vi "Dashboard Main.vi"() -> ()   [LabVIEW 2018]
uses:
  <vilib>/Utility/miscctls.llb/LVRowAndColumnTypeDef.ctl
  <vilib>/event_ctls.llb/eventvkey.ctl
  <vilib>/Rock Robotics/Network Tables/NT Read Numeric Array.vi
  <vilib>/Rock Robotics/Network Tables/NT Write Boolean.vi
  <vilib>/Rock Robotics/Network Tables/NT Read Boolean.vi
  <vilib>/Rock Robotics/WPI/Dashboard/WPI_DashboardLogging Global.vi
panel:
  in  "Camera Settings Right":T1={"Frame Rate"=30, "Compression"=30, "Size"=1, "DB Camera Config"=FALSE} {"Frame Rate" scale=1.0..30.0; "Compression" scale=100.0..-1.0; "Size" items=["640x480", "320x240", "160x120"]}
  in  "Camera Name Right":string(combo)="No Camera Selection"
  out "Camera Perf":string
  in  "Camera Settings":T1={"Frame Rate"=30, "Compression"=30, "Size"=1, "DB Camera Config"=FALSE} {"Frame Rate" scale=1.0..30.0; "Compression" scale=100.0..-1.0; "Size" items=["640x480", "320x240", "160x120"]}
  in  "TCP":refnum<k5>
  in  "Rec Mode":enum32{"Stop", "Record", "Playback"}(radio)
  out "Robot IP":string
  out "Image Message":string="Timeout in Camera Communications"
  in  "Dashboard Tab":T2(tab)
  in  "Select Auto":string(combo)="Select Autonomous ..."
  out "NT Connection":bool
  out "MotorChart R":cluster{"Numeric":dbl, "Numeric":dbl}(graph)
  out "MotorChart L":cluster{"Numeric":dbl, "Numeric":dbl}(graph)
  out "MotorSliders R":cluster{"MotorSlide1":dbl, "MotorSlide2":dbl} {"MotorSlide2" scale=-1.0..1.0 scale format="%#_2e"; "MotorSlide1" scale=-1.0..1.0 scale format="%#_2e"}
  out "MotorSliders L":cluster{"MotorSlide1":dbl, "MotorSlide2":dbl} {"MotorSlide2" scale=-1.0..1.0 scale format="%#_2e"; "MotorSlide1" scale=-1.0..1.0 scale format="%#_2e"}
  out "Gyro":dbl(knob) scale=0.0..360.0
  out "JS1 Z":dbl(slide) scale=-1.0..1.0 scale format="%#_2e"
  out "JS1 Graph":cluster{"X":dbl, "Y":dbl}[](graph)
  out "JS1 Buttons":T3
  out "JS2 Z":dbl(slide) scale=-1.0..1.0 scale format="%#_2e"
  out "JS2 Graph":cluster{"X":dbl, "Y":dbl}[](graph)
  out "JS2 Buttons":T3
  out "Mode":T4(ring)=enum."Auto Disabled"
  out "Right Camera Perf":cluster{"Bandwidth (Mbps)":dbl, "FPS":dbl}
  out "Camera Image Right":T5(plugin-control)
  in  "DB/String 9":string
  in  "DB/String 8":string
  in  "DB/String 7":string
  in  "DB/String 6":string
  in  "DB/String 5":string
  in  "DB/String 4":string
  in  "DB/String 3":string
  in  "DB/String 2":string
  in  "DB/String 1":string
  in  "DB/String 0":string
  in  "DB/Slider 0":dbl(slide) scale=0.0..5.0
  in  "DB/Slider 1":dbl(slide) scale=0.0..5.0
  in  "DB/Slider 2":dbl(slide) scale=0.0..5.0
  in  "DB/Slider 3":dbl(slide) scale=0.0..5.0
  out "DB/LED 3":bool
  out "DB/LED 2":bool
  out "DB/LED 1":bool
  out "DB/LED 0":bool
  in  "DB/Button 3":bool
  in  "DB/Button 2":bool
  in  "DB/Button 1":bool
  in  "DB/Button 0":bool caption="New Name"
  in  "Robot Front":bool
  in  "Calibrate?":bool
  out "ElevEncPos":dbl
  out "ElevBasePos":string
  out "PickUp/DropOff":string
  out "SwerveMode":string
  out "Yaw":dbl
  out "Hatch Position":bool
  in  "Test Slider":dbl(slide) scale=0.0..100.0 scale format="%#_3g"
  in  "On/Off":bool caption="Solenoid"
  in  "Test Name":u16(ring) items=["Select the test to run..."]
  in  "Test Tree":string(tree)
  in  "Motor":cluster{"Value":dbl, "Enable":bool} {"Value" scale=-1.0..1.0 scale format="%#_3g"}
  out "Progress":T6 {"Test Progress" scale=0.0..100.0}
  in  "Rev/Fwd":cluster{"Forward":bool, "Reverse":bool}
  in  "Test Ring":u16(ring) items=["Monochrome", "Color"]
  out "Cmd Status":string
  in  "Execute Command":bool
  in  "Command Params":string[][](table)
  in  "Command Selection":i32(listbox)
  in  "CheckList":i32(listbox)
  out "Tree":string(tree)
  out "Camera Image":T5(plugin-control)
  out "Background":bool
  in  "Camera Name":string(combo)="No Camera Selection"
  # "HW"
  # "HW"
  # "Joysticks"
  # "Drive Motors"
  # "Front"
  # "Right"
  # "Left"
  # "Back"
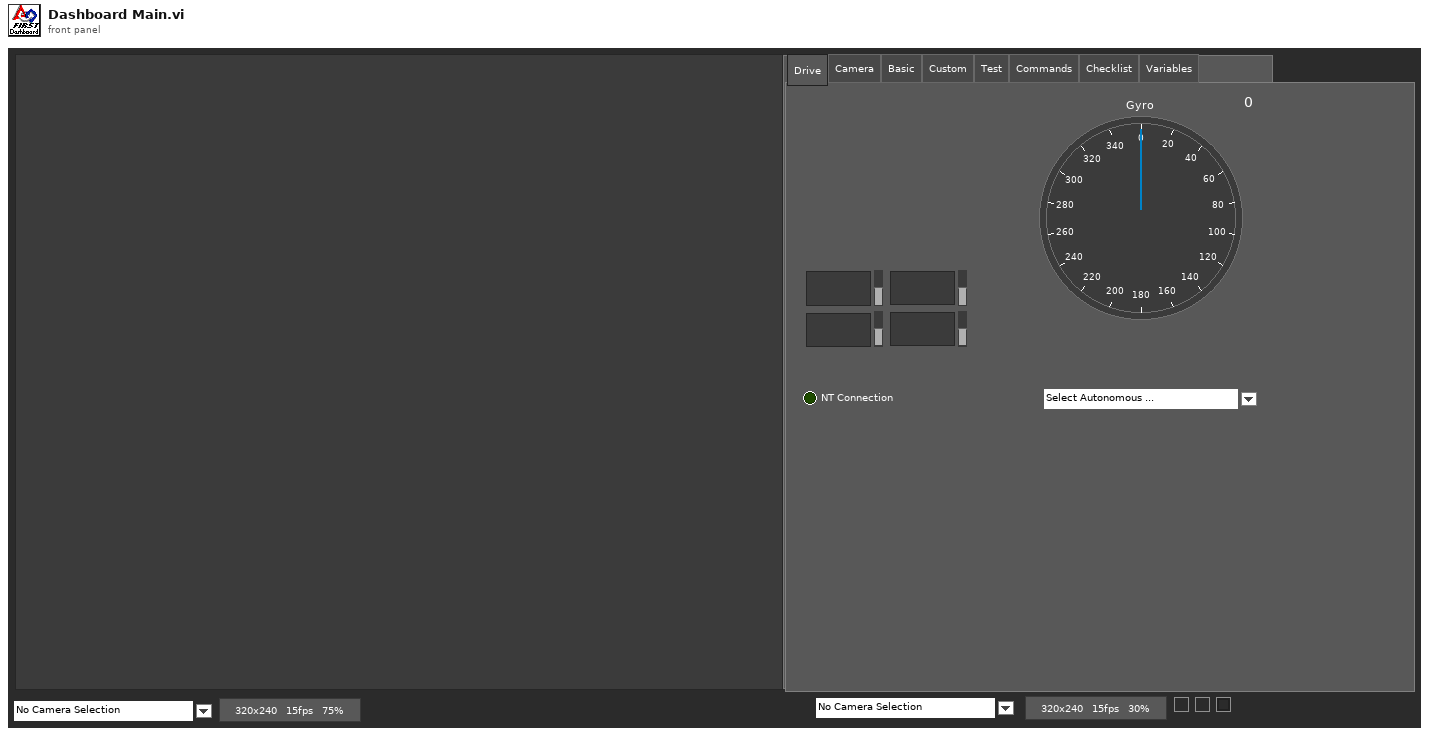
[diagram p1: front panel]
types:
  T1 = cluster{"Frame Rate":i32, "Compression":i32, "Size":u16, "DB Camera Config":bool}
  T2 = enum32{"Drive", "Camera", "Basic", "Custom", "Test", "Commands", "Checklist", "Variables"}
  T3 = cluster{bool, bool, bool, bool, bool, bool, bool, bool, bool, bool, bool, bool}
  T4 = enum8{"Tele-Op Disabled", "Tele-Op Enabled", "Auto Disabled", "Auto Enabled", "Test Disabled", "Test Enabled", "Disconnected", "No Code", "E-Stop"}
  T5 = typedef "IMAQ Image.ctl" = refnum<image>
  T6 = cluster{"Test Progress":u8, "Test Progress Text":string}
  T7 = cluster{"Save Path":path, "Interval (s)":dbl, "Keep":i32}
  T8 = typedef "Image Type" = u32
  T9 = cluster{"IDs":cluster{"RPC field ID":u16, "Unique ID":u16}, "String":string}
  T10 = cluster{"Error Strings":string, "Disable Counts":cluster{u16, u16}, "Rail Faults":cluster{u16, u16, u16}, "Robot IP":string, "DB Mode":u8, "Event Info":cluster{"Name":string, "Type":u8, "Number":u16, "Replay":u8}}
  T11 = cluster{"Storage":cluster{"Disk Free":u64, "RAM Block":u32, "RAM free":u32}, "CPU Utilization":cluster{"CPU % ISR":sgl, "CPU % Time Crit":sgl, "CPU % Timed Str":sgl, "CPU % High":sgl, "CPU % Above":sgl, "CPU % Normal":sgl, "CPU % Low":sgl}, "CAN":cluster{"% Bus Utilization":sgl, "Bus Off Cnt":u32, "TX_FIFO Full Cnt":u32, "Receive Error Cnt":u8, "Transmit Error Cnt":u8}, "HID":cluster{"HID Outputs":u32, "Rumble Low":u16, "Rumble High":u16}[]}
  T12 = cluster{"Status bits":cluster{"Test Mode":bool, "Autonomous":bool, "Enabled":bool, "Code Start":bool, "Brownout":bool, "Reserved 2":bool, "Reserved 3":bool, "E-Stop":bool}, "Code Trace":cluster{"Disabled":bool, "TeleOp":bool, "Auto":bool, "Test":bool}, "Controller Type":enum16{"unknown", "cRIO", "roboRio"}, "Code?":enum16{"unknown", "noCode", "code"}, "Battery V":dbl}
  T13 = cluster{"Control Bits":cluster{"TestMode":bool, "Autonomous":bool, "Enabled":bool, "FMS Present":bool, bool, bool, bool, "E-Stop":bool}, "Team Station ":u8, "Countdown":sgl, "Joystick Values":cluster{"Axes":dbl[], "Buttons":bool[], "POVs":i16[]}[]}
  T14 = cluster{"Axes":dbl[], "Buttons":bool[], "POVs":i16[]}[]
  T15 = cluster{"Axes":dbl[], "Buttons":bool[], "POVs":i16[]}
  T16 = cluster{"Buttons[0]":bool, "Buttons[1]":bool, "Buttons[2]":bool, "Buttons[3]":bool, "Buttons[4]":bool, "Buttons[5]":bool, "Buttons[6]":bool, "Buttons[7]":bool, "Buttons[8]":bool, "Buttons[9]":bool, "Buttons[10]":bool, "Buttons[11]":bool}
  T17 = cluster{"Camera Image":refnum<vi>, "Dashboard Tab":refnum<vi>, "Background":refnum<vi>, "Rec Mode":refnum<vi>, "Test Slider":refnum<vi>, "On/Off ":refnum<vi>, "Test Ring":refnum<vi>, "Rev/Fwd":refnum<vi>, "Test Name":refnum<vi>, "Motor":refnum<vi>, "Progress":refnum<vi>, "CheckList":refnum<vi>, "Tree":refnum<vi>, "Test Tree":refnum<vi>, "Command Params":refnum<vi>, "Command Selection":refnum<vi>, "Execute Command":refnum<vi>, "Cmd Status":refnum<vi>, "Camera Settings":refnum<vi>, "Camera Name":refnum<vi>, "Camera Perf":refnum<vi>, "Camera Settings Right":refnum<vi>, "Camera Name Right":refnum<vi>, "Camera Image Right":refnum<vi>}
  T18 = cluster{"Global Rectangle":i32[], "Contours":cluster{"Contour Type":u32, "ROI Type":u32, "Points":i32[]}[]}
  T19 = cluster{"Camera Name":string, string, "Saved DB Images Info":cluster{"Save Path":path, "Interval (s)":dbl, "Keep":i32}}
  T20 = cluster{"Camera Name Right":string, string, "Saved DB Images Info":cluster{"Save Path":path, "Interval (s)":dbl, "Keep":i32}}
  T21 = cluster{"Operation":enum16{"Update", "Clear"}, "Color Box":u32}[]
  T22 = typedef "eventvkey.ctl" = enum16{"ASCII", "Enter", "Return", "Shift", "Ctrl", "Alt", "Cmd", "Opt", "Caps", "NumLock", "Clear", "Break", "Up", "Down", "Left", "Right", "Insert", "Delete", "Home", "End", "PageUp", "PageDown", "Escape", "Help", "Pause", "ScrollLock", "F1", "F2", "F3", "F4", "F5", "F6", "F7", "F8", "F9", "F10", "F11", "F12", "F13", "F14", "F15", "F16", "F17", "F18", "F19", "F20", "F21", "F22", "F23", "F24", "Play", "VolumeUp", "VolumeDown", "Mute", "Two Byte Char"}
  T23 = cluster{"Image Size":bool, "Image Type":bool, "Pixel Value":bool, "ROI Information":bool, "Zoom Factor":bool}
  T24 = cluster{"Operation":enum16{"Update", "Clear"}, "Color Box":u32}
  T25 = typedef "LVRowAndColumnTypeDef.ctl" = cluster{"Row":i32, "Column":i32}
  T26 = cluster{"Shift":bool, "Ctrl":bool, "Alt":bool, "Cmd":bool, "Opt":bool}
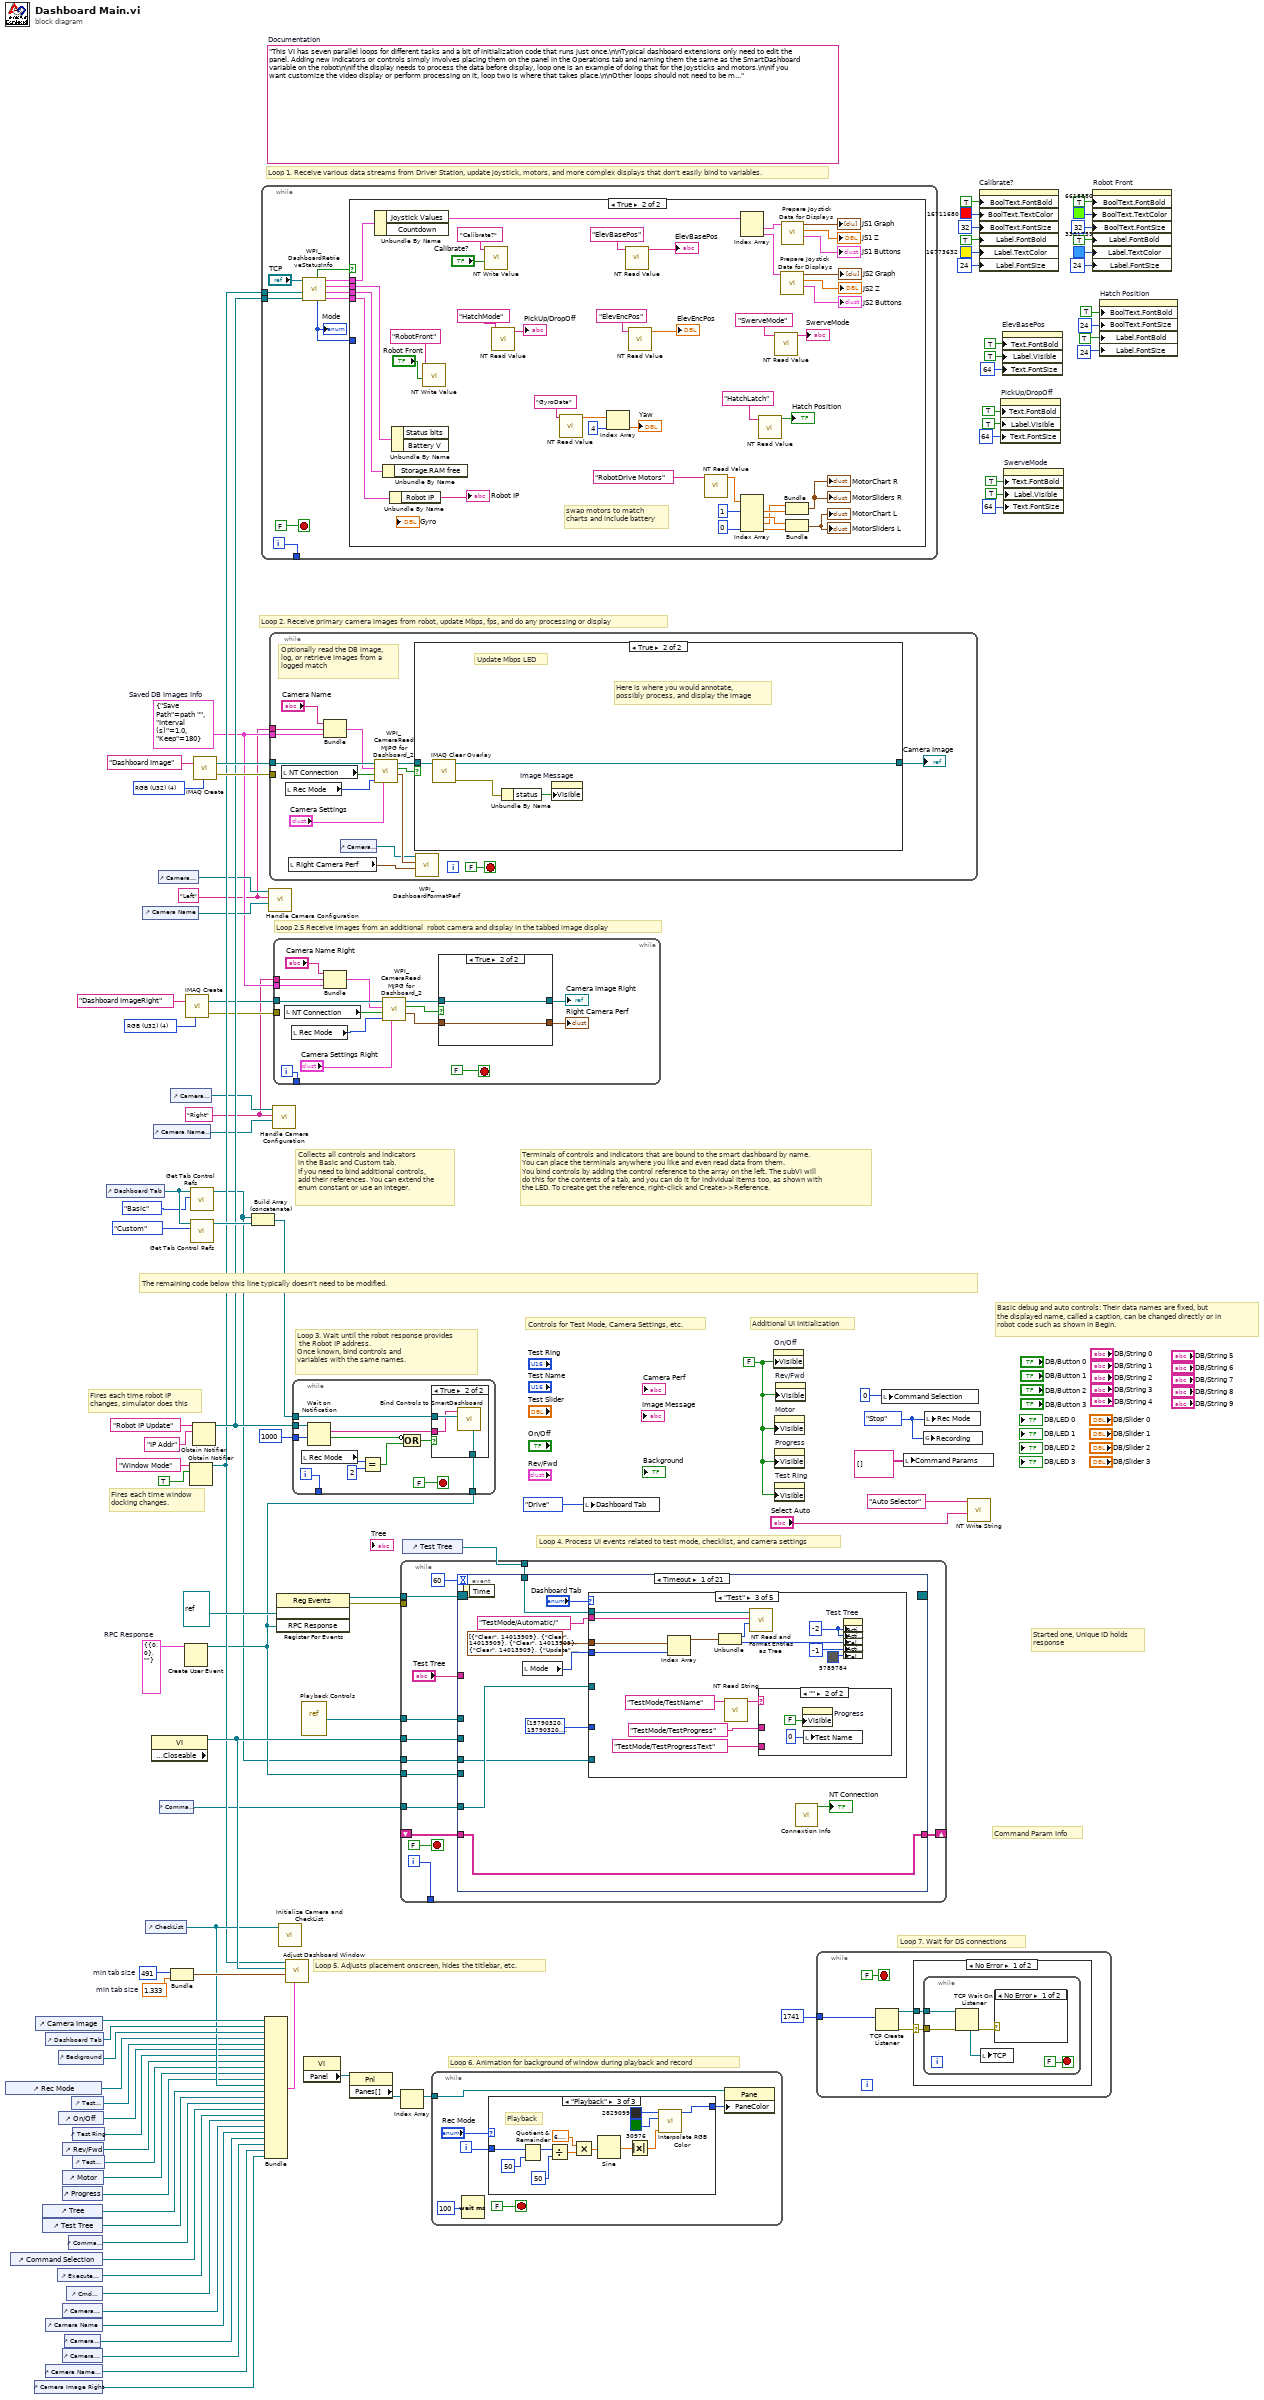
[diagram p0: block diagram]
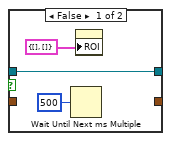
[diagram p2: hidden frame]
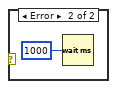
[diagram p3: hidden frame]
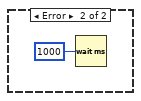
[diagram p4: hidden frame]
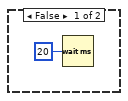
[diagram p5: hidden frame]
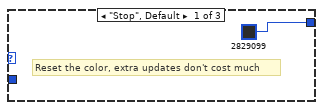
[diagram p6: hidden frame]
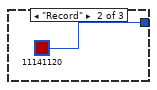
[diagram p7: hidden frame]
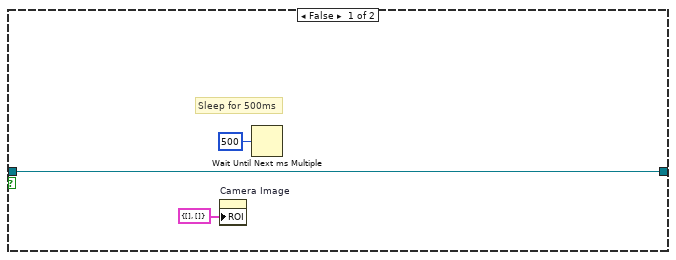
[diagram p9: hidden frame]
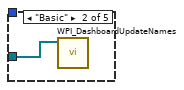
[diagram p11: hidden frame]
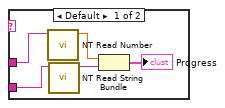
[diagram p12: hidden frame]
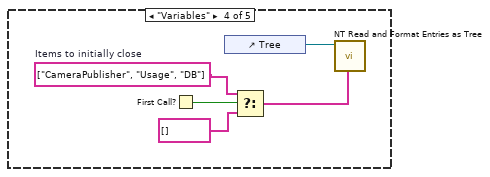
[diagram p13: hidden frame]
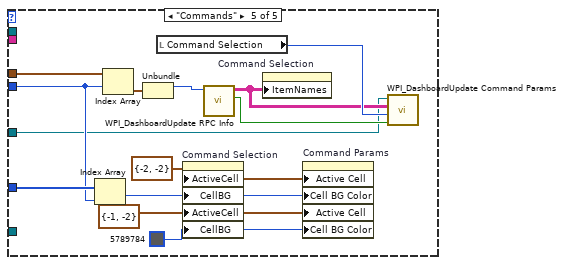
[diagram p14: hidden frame]
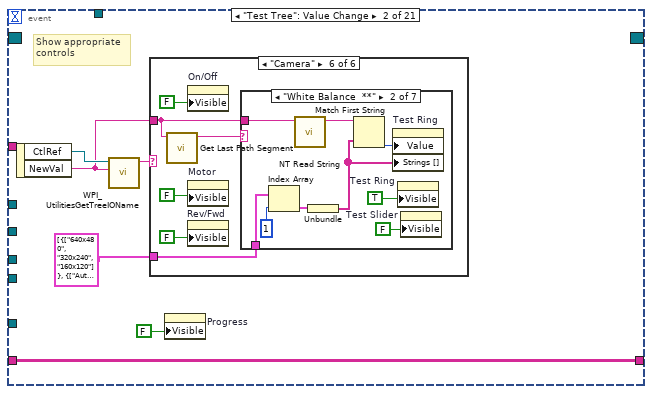
[diagram p15: hidden frame]
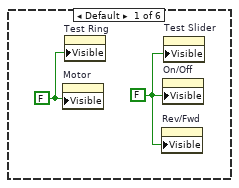
[diagram p16: hidden frame]
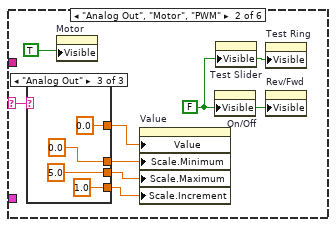
[diagram p17: hidden frame]
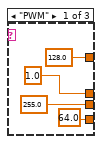
[diagram p18: hidden frame]
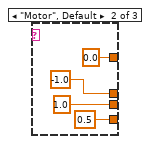
[diagram p19: hidden frame]
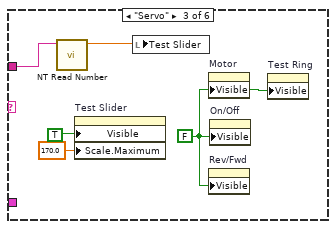
[diagram p20: hidden frame]
diagram:
  w28 = T7 {"Save Path"=path "", "Interval (s)"=1.0, "Keep"=180}  # Saved DB Images Info
  w27 = "Right"
  w26 = "Left"
  w38 = T8 4 items=["Grayscale (U8)", "Grayscale (I16)", "Grayscale (SGL)", "Complex (CSG)", "RGB (U32)", "HSL (U32)", "RGB (U64)"] ("Image Type")
  w54 = T9 {"IDs"={"RPC field ID"=0, "Unique ID"=0}, "String"=""}  # RPC Response
  w77 = 491  # min tab size
  w76 = 1.333  # min tab size
  w84 = enum32{"Stop", "Record", "Playback"}."Stop" ("Rec Mode")
  w61 = FALSE ("Visible")
  (unwired) "This VI has seven parallel loops for different tasks and a bit of initialization code that runs just once.\n\nTypical dashboard extensions only need to edit the panel. Adding new indicators or controls simply involves placing them on the panel in the Operations tab and naming them the same as the SmartDashboard variable on the robot\n\nIf the display needs to process the data before display, loop one is an example of doing that for the joysticks and motors.\n\nIf you want customize the video display or perform processing on it, loop two is where that takes place.\n\nOther loops should not need to be modified. They are pretty standard, and document the task they perform."  # Documentation
  w101 = T8 4 items=["Grayscale (U8)", "Grayscale (I16)", "Grayscale (SGL)", "Complex (CSG)", "RGB (U32)", "HSL (U32)", "RGB (U64)"] ("Image Type")
  # "Loop 2.5 Receive images from an additional  robot camera and display in the tabbed image display"
  # "Command Param Info"
  # "Started one, Unique ID holds\nresponse"
  # "Loop 7. Wait for DS connections"
  # "Basic debug and auto controls: Their data names are fixed, but\nthe displayed name, called a caption, can be changed directly or in\nrobot code such as shown in Begin."
  # "Controls for Test Mode, Camera Settings, etc."
  # "Additional UI Initialization"
  # "Loop 6. Animation for background of window during playback and record"
  # "Fires each time robot IP\nchanges, simulator does this"
  # "Fires each time window\ndocking changes."
  # "Collects all controls and indicators\nin the Basic and Custom tab.\nIf you need to bind additional controls,\nadd their references. You can extend the\nenum constant or use an integer."
  # "The remaining code below this line typically doesn't need to be modified."
  # "Loop 4. Process UI events related to test mode, checklist, and camera settings"
  # "Terminals of controls and indicators that are bound to the smart dashboard by name.\nYou can place the terminals anywhere you like and even read data from them.\nYou bind controls by adding the control reference to the array on the left. The subVI will\ndo this for the contents of a tab, and you can do it for individual items too, as shown with\nthe LED. To create get the reference, right-click and Create>>Reference."
  # "Loop 3. Wait until the robot response provides\n the Robot IP address.\nOnce known, bind controls and\nvariables with the same names."
  # "Loop 5. Adjusts placement onscreen, hides the titlebar, etc."
  # "Loop 1. Receive various data streams from Driver Station, update joystick, motors, and more complex displays that don't easily bind to variables."
  # "Loop 2. Receive primary camera images from robot, update Mbps, fps, and do any processing or display"
  n1 = control-ref of="Rec Mode"() -> (w67:refnum<vi>)
  n2 = control-ref of="Command Selection"() -> (w53:refnum<vi>)
  n3 = control-ref of="Camera Image Right"() -> (w31:refnum<vi>)
  n4 = control-ref of="Camera Image"() -> (w79:refnum<vi>)
  n5 = control-ref of="Tree"() -> (w71:refnum<vi>)
  n6 = control-ref of="Test Tree"() -> (w70:refnum<vi>)
  n7 = control-ref of="Dashboard Tab"() -> (w78:refnum<vi>)
  n8 = control-ref of="Camera Name"() -> (w44:refnum<vi>)
  n9 = control-ref of="Camera Name Right"() -> (w32:refnum<vi>)
  n10 = control-ref of="Execute Command"() -> (w55:refnum<vi>)
  n11 = control-ref of="Background"() -> (w74:refnum<vi>)
  n12 = control-ref of="On/Off"() -> (w65:refnum<vi>)
  n13 = control-ref of="Progress"() -> (w62:refnum<vi>)
  n14 = control-ref of="Camera Settings"() -> (w45:refnum<vi>)
  n15 = control-ref of="Camera Settings Right"() -> (w33:refnum<vi>)
  n16 = control-ref of="Rev/Fwd"() -> (w63:refnum<vi>)
  n17 = control-ref of="Motor"() -> (w68:refnum<vi>)
  n18 = control-ref of="Camera Perf"() -> (w43:refnum<vi>)
  n19 = control-ref of="Cmd Status"() -> (w49:refnum<vi>)
  n20 = control-ref of="Command Params"() -> (w56:refnum<vi>)
  n21 = control-ref of="Test Slider"() -> (w66:refnum<vi>)
  n22 = control-ref of="Test Ring"() -> (w64:refnum<vi>)
  n23 = control-ref of="Test Name"() -> (w69:refnum<vi>)
  n24 = control-ref of="Dashboard Tab"() -> (w82:refnum<vi>)
  n25 = control-ref of="Camera Name"() -> (w46:refnum<vi>)
  n26 = control-ref of="CheckList"() -> (w72:refnum<vi>)
  n27 = property class="VI" props=["Front Panel.Closeable"]() -> (reference out=w83:refnum<vi>)  [unwired: 2 in, 2 out]
  n28 = control-ref of="Camera Name Right"() -> (w34:refnum<vi>)
  n29 = control-ref of="Camera Settings"() -> (w47:refnum<vi>)
  n30 = control-ref of="Command Params"() -> (w48:refnum<vi>)
  n31 = control-ref of="Camera Settings Right"() -> (w35:refnum<vi>)
  n32 = Bundle("min tab size"=w77, "min tab size"=w76) -> (w75:cluster{"min tab size":i32, "min tab size":dbl})  [unwired: 1 in]
  n33 = Create User Event(user event datatype=w54) -> (user event=w50:refnum<user-event>)  [unwired: 1 in, 1 out]
  n34 = call "IMAQ Create"("Image Name"="Dashboard ImageRight", "Image Type"=w38) -> ("New Image"=w37:T5, "error out"=w36:errorcluster)  [unwired: 2 in, 1 out]
  n35 = Obtain Notifier(name (unnamed)="Window Mode", notification data type=TRUE) -> (notifier out=w59:refnum<notifier>)  [unwired: 2 in, 2 out]
  n36 = call <vilib>:"Get Tab Control Refs.vi"("Page Index"=T2."Basic" ("Dashboard Tab"), "TabControl in"=w82) -> ("ControlsOnPage"=w42:refnum<vi>[])  [unwired: 9 in]
  n37 = call <vilib>:"Get Tab Control Refs.vi"("Page Index"=T2."Custom" ("Dashboard Tab"), "TabControl in"=w82) -> ("ControlsOnPage"=w81:refnum<vi>[])  [unwired: 9 in]
  n38 = Obtain Notifier(name (unnamed)="Robot IP Update", notification data type="IP Addr" ("name (unnamed)")) -> (notifier out=w60:refnum<notifier>)  [unwired: 2 in, 2 out]
  n39 = call "IMAQ Create"("Image Name"="Dashboard Image", "Image Type"=w101) -> ("New Image"=w99:T5, "error out"=w98:errorcluster)  [unwired: 2 in, 1 out]
  n40 = Build Array (concatenate)(w42, w81) -> (w80:refnum<vi>[])
  n41 = while {
    tunnel: [w111] -> _
    tunnel: w60 -> [w106]
    tunnel: w59 -> [w103]
    i -> [w111]
    stop <- FALSE stop-if-true
    n42 = call <vilib>:"WPI_DashboardRetrieveStatusInfo.vi"("Binding Refnum"=w106, "Window Mode Notifier"=w103, "TCP Cnx"="TCP") -> ("Power and Errors"=w107:T10, "Robot Metrics"=w109:T11, "Status Info"=w110:T12, "Control Info"=w108:T13, "Robot Mode"=w105:T4, "Process?"=w102:bool)  [unwired: 3 in]
    "Mode" <- w105
    n43 = case shown="True" w102 {
      tunnel: w110 -> [_ w155]
      tunnel: w109 -> [_ w154]
      tunnel: w108 -> [_ w153]
      tunnel: w107 -> [_ w152]
      tunnel: w105 -> [_ _]
      frame False {
        n44 = Wait (ms)(milliseconds to wait=u32 20) -> ()  [unwired: 1 out]
      }
      frame True {
        # "swap motors to match\ncharts and include battery"
        n45 = Unbundle By Name(w153) -> ("Joystick Values"=w143:T14)  [unwired: 1 out]
        n46 = Unbundle By Name(w154) -> ()  [unwired: 1 out]
        n47 = Unbundle By Name(w152) -> ("Robot IP"=→"Robot IP":string)
        n48 = Unbundle By Name(w155) -> ()  [unwired: 2 out]
        n49 = call-poly <vilib>:"NT Write Value.vi"("Boolean"="Robot Front", "Name"="RobotFront") -> ()  [unwired: 9 in, 1 out]
        n50 = call-poly <vilib>:"NT Write Value.vi"("Boolean"="Calibrate?", "Name"="Calibrate?") -> ()  [unwired: 9 in, 1 out]
        n51 = call-poly <vilib>:"NT Read Value.vi"("Name"="HatchMode") -> ("String"=→"PickUp/DropOff":string)  [unwired: 9 in, 1 out]
        n52 = call-poly <vilib>:"NT Read Value.vi"("Name"="GyroData") -> ("Numeric Array"=w120:dbl[])  [unwired: 9 in, 1 out]
        n53 = Index Array(array=w120, index=4) -> (element=→"Yaw":dbl)
        n54 = call-poly <vilib>:"NT Read Value.vi"("Name"="ElevBasePos") -> ("String"=→"ElevBasePos":string)  [unwired: 9 in, 1 out]
        n55 = call-poly <vilib>:"NT Read Value.vi"("Name"="ElevEncPos") -> ("Numeric"=→"ElevEncPos":dbl)  [unwired: 9 in, 1 out]
        n56 = call-poly <vilib>:"NT Read Value.vi"("Name"="RobotDrive Motors") -> ("Numeric Array"=w133:dbl[])  [unwired: 9 in, 1 out]
        n57 = Index Array(array=w143) -> (element #1=w142:T15, element #2=w138:T15)  [unwired: 2 in]
        n58 = Index Array(array=w133, index #1=1, index #4=0) -> (element #1=w147:dbl, element #2=w148:dbl, element #3=w146:dbl, element #4=w151:dbl)  [unwired: 2 in]
        n59 = call-poly <vilib>:"NT Read Value.vi"("Name"="HatchLatch") -> ("Boolean"=→"Hatch Position":bool)  [unwired: 9 in, 1 out]
        n60 = call-poly <vilib>:"NT Read Value.vi"("Name"="SwerveMode") -> ("String"=→"SwerveMode":string)  [unwired: 9 in, 1 out]
        n61 = call "Prepare Joystick Data for Displays.vi"("Joystick Values"=w138) -> ("Buttons"=→"JS2 Buttons":T16, "Z Axis"=→"JS2 Z":dbl, "Cartesian Data"=→"JS2 Graph":cluster{"X axis":dbl, "X axis":dbl}[])  [unwired: 8 in]
        n62 = call "Prepare Joystick Data for Displays.vi"("Joystick Values"=w142) -> ("Buttons"=→"JS1 Buttons":T16, "Z Axis"=→"JS1 Z":dbl, "Cartesian Data"=→"JS1 Graph":cluster{"X axis":dbl, "X axis":dbl}[])  [unwired: 8 in]
        n63 = Bundle("Numeric"=w146, "Numeric"=w147) -> (→"MotorChart R" →"MotorSliders R":cluster{"Numeric":dbl, "Numeric":dbl})  [unwired: 1 in]
        n64 = Bundle("Numeric"=w148, "Numeric"=w151) -> (→"MotorChart L" →"MotorSliders L":cluster{"Numeric":dbl, "Numeric":dbl})  [unwired: 1 in]
      }
    }
  }
  n65 = Bundle("Camera Image"=w79, "Dashboard Tab"=w78, "Background"=w74, "Rec Mode"=w67, "Test Slider"=w66, "On/Off"=w65, "Test Ring"=w64, "Rev/Fwd"=w63, "Test Name"=w69, "Motor"=w68, "Progress"=w62, "CheckList"=w72, "Tree"=w71, "Test Tree"=w70, "Command Params"=w56, "Command Selection"=w53, "Execute Command"=w55, "Cmd Status"=w49, "Camera Settings"=w45, "Camera Name"=w44, "Camera Perf"=w43, "Camera Settings Right"=w33, "Camera Name Right"=w32, "Camera Image Right"=w31) -> (w73:T17)  [unwired: 1 in]
  n66 = call "Handle Camera Configuration.vi"("CameraNameRef"=w46, "Display Name"=w26, "ClusterRef"=w47) -> ()  [unwired: 9 in]
  n67 = while {
    tunnel: w99 -> [w169]
    tunnel: w98 -> [_]
    tunnel: w28 -> [w162]
    tunnel: w26 -> [w159]
    stop <- FALSE stop-if-true
    # "Optionally read the DB image,\nlog, or retrieve images from a\nlogged match"
    n68 = local read "NT Connection"() -> (w163:bool)
    n69 = local read "Rec Mode"() -> (w166:enum32{"Stop", "Record", "Playback"})
    n70 = local read "Right Camera Perf"() -> (w157:cluster{"Bandwidth (Mbps)":dbl, "FPS":dbl})
    n71 = Bundle("Camera Name"="Camera Name", w159, "Saved DB Images Info"=w162) -> (w161:T19)  [unwired: 1 in]
    n72 = control-ref of="Camera Perf"() -> (w156:refnum<vi>)
    n73 = call <vilib>:"WPI_CameraRead MJPG for Dashboard_2.vi"("Camera Settings"="Camera Settings", "Rec Mode"=w166, "NT Connection"=w163, "Capture Info"=w161, "Image in"=w169) -> ("perf info"=w158:cluster{"Bandwidth (Mbps)":dbl, "fps":dbl}, "Active"=w167:bool, "Image\\ out"=w168:T5)  [unwired: 4 in]
    n74 = case shown="True" w167 {
      tunnel: w168 -> [w172 w175]
      tunnel: [w172 w174] -> w164
      frame False {
        # "Sleep for 500ms"
        n75 = property on="Camera Image" class="ImageControl"("ROI"=T18 {"Global Rectangle"=[], "Contours"=[]}) -> ()  [unwired: 2 in, 2 out]
        n76 = Wait Until Next ms Multiple(millisecond multiple=u32 500) -> ()  [unwired: 1 out]
      }
      frame True {
        # "Here is where you would annotate,\npossibly process, and display the image"
        # "Update Mbps LED"
        n77 = call "IMAQ Clear Overlay"("Image"=w175) -> ("error out"=w176:errorcluster, "Image Out"=w174:T5)  [unwired: 2 in, 7 out]
        n78 = Unbundle By Name(w176) -> ("status"=w177:bool)
        n79 = property on="Image Message" class="Str"("Visible"=w177) -> ()  [unwired: 2 in, 2 out]
      }
    }
    "Camera Image" <- w164
    n80 = call <vilib>:"WPI_DashboardFormatPerf.vi"("Right Camera Perf"=w157, "Performance"=w158, "String in"=w156) -> ()  [unwired: 9 in]
  }
  n81 = call "Handle Camera Configuration.vi"("CameraNameRef"=w34, "Display Name"=w27, "ClusterRef"=w35) -> ()  [unwired: 9 in]
  n82 = while {
    tunnel: w37 -> [w192]
    tunnel: w36 -> [_]
    tunnel: [w187] -> _
    tunnel: w28 -> [w183]
    tunnel: w27 -> [w180]
    i -> [w187]
    stop <- FALSE stop-if-true
    n83 = local read "NT Connection"() -> (w184:bool)
    n84 = local read "Rec Mode"() -> (w191:enum32{"Stop", "Record", "Playback"})
    n85 = Bundle("Camera Name Right"="Camera Name Right", w180, "Saved DB Images Info"=w183) -> (w182:T20)  [unwired: 1 in]
    n86 = call <vilib>:"WPI_CameraRead MJPG for Dashboard_2.vi"("Camera Settings"="Camera Settings Right", "Rec Mode"=w191, "NT Connection"=w184, "Capture Info"=w182, "Image in"=w192) -> ("perf info"=w178:cluster{"Bandwidth (Mbps)":dbl, "fps":dbl}, "Active"=w186:bool, "Image\\ out"=w189:T5)  [unwired: 4 in]
    n87 = case shown="True" w186 {
      tunnel: w189 -> [w194 w197]
      tunnel: [w194 w197] -> w185
      tunnel: [_ w196] -> w179
      tunnel: w178 -> [_ w196]
      frame False {
        n88 = Wait Until Next ms Multiple(millisecond multiple=u32 500) -> ()  [unwired: 1 out]
        n89 = property on="Camera Image Right" class="ImageControl"("ROI"=T18 {"Global Rectangle"=[], "Contours"=[]}) -> ()  [unwired: 2 in, 2 out]
      }
      frame True {
      }
    }
    "Camera Image Right" <- w185
    "Right Camera Perf" <- w179
  }
  n90 = register-events(refnum<vi> refnum, w50) -> (reference out=w88:refnum<event-registration>, error out=w87:errorcluster)  [unwired: 2 in]
  n91 = call "Initialize Camera and CheckList.vi"("ListBox in"=w72) -> ()  [unwired: 11 in]
  n92 = call "Adjust Dashboard Window.vi"("Sizing Refnums"=w73, "Size Constraints"=w75, "VI"=w83, "WIn Mode"=w59) -> ()  [unwired: 8 in]
  n93 = while {
    tunnel: w80 -> [w209]
    tunnel: w60 -> [w207]
    tunnel: [w205] -> _
    tunnel: u32 1000 ("milliseconds to wait") -> [w204]
    tunnel: w50 -> [w198]
    i -> [w205]
    stop <- FALSE stop-if-true
    n94 = local read "Rec Mode"() -> (w200:enum32{"Stop", "Record", "Playback"})
    n95 = Wait on Notification(notifier=w207, timeout in ms (-1)=w204) -> (notification=w206:string, timed out?=w202:bool)  [unwired: 2 in, 2 out]
    n96 = Equal?(x=w200, y=u16 2 ("Rec Mode")) -> (x = y?=w201:bool)
    n97 = Compound Arithmetic op=OR(invert w202, w201) -> (w203:bool)
    n98 = case shown="True" w203 {
      tunnel: w209 -> [_ w212]
      tunnel: w206 -> [_ w211]
      tunnel: w198 -> [_ w210]
      frame False {
      }
      frame True {
        n99 = call <vilib>:"Bind Controls to SmartDashboard.vi"("RPC ref"=w210, "Bound Control Refs"=w212, "Server IP Address"=w211) -> ()  [unwired: 9 in]
      }
    }
  }
  n100 = vi-ref "Playback Controls.vi"() -> (w89:refnum<vi>)
  n101 = property class="VI"() -> ("Panel"=w91:refnum<vi>)  [unwired: 2 in, 2 out]
  n102 = property class="Pnl"(reference=w91) -> ("Panes[]"=w92:refnum<vi>[])  [unwired: 1 in, 2 out]
  n103 = Index Array(array=w92) -> (element=w90:refnum<vi>)  [unwired: 1 in]
  n104 = control-ref of="Test Tree"() -> (w93:refnum<vi>)
  n105 = while {
    tunnel: [w222] -> _
    tunnel: w93 -> [w221]
    tunnel: w89 -> [w220]
    tunnel: w88 -> [w219]
    tunnel: w87 -> [_]
    tunnel: w83 -> [w218]
    tunnel: w50 -> [w217]
    tunnel: w48 -> [w216]
    shift-right: [w215] -> _
    shift-left: _ -> [w214]
    tunnel: w42 -> [w213]
    i -> [w222]
    stop <- FALSE stop-if-true
    n106 = event shown="[0] Timeout" {
      selector: w219 -> [_ _ _ _ _ _ _ _ _ _ _ _ _ _ _ _ _ _ _ _ _]
      dyn-events: [_ _ _ _ _ _ _ _ _ _ _ _ _ _ _ _ w482 _ _ _ _] -> _
      timeout: u32 60 ("milliseconds to wait") -> [_ _ _ _ _ _ _ _ _ _ _ _ _ _ _ _ _ _ _ _ _]
      tunnel: w221 -> [w234 _ _ _ _ _ _ _ _ _ _ _ _ _ _ _ _ _ _ _ _]
      tunnel: "Test Tree" -> [_ _ _ _ _ _ _ _ _ _ _ w449 w457 w459 w463 w471 _ _ _ _ _]
      tunnel: w220 -> [_ _ _ _ _ _ _ _ _ _ _ _ _ _ _ _ w484 _ w502 _ _]
      tunnel: w218 -> [_ _ _ _ _ _ _ _ _ _ _ _ _ _ _ _ w480 _ _ _ _]
      tunnel: w217 -> [_ _ _ _ _ _ _ _ _ _ _ _ _ _ _ _ w478 _ _ _ _]
      tunnel: w216 -> [w229 _ _ _ _ _ w400 _ _ _ _ _ _ _ _ _ _ _ _ _ _]
      tunnel: [w228 w277 w379 w384 w393 w397 w398 w407 w417 w424 w436 w448 w455 w458 w462 w470 w477 w497 w499 w503 w516] -> w215
      tunnel: w214 -> [w228 w277 w379 w384 w393 w397 w398 _ _ w424 w436 w448 w455 w458 w462 w470 w477 w497 w499 w503 w516]
      tunnel: w213 -> [w226 _ _ _ _ _ _ _ _ _ _ _ _ _ _ _ _ _ _ _ _]
      event Timeout {
        n107 = event-data() -> ()  [unwired: 1 in, 1 out]
        n108 = local read "Mode"() -> (w231:T4)
        n109 = case shown="\"Test\"" "Dashboard Tab" {
          tunnel: w234 -> [_ _ w250 _ _]
          tunnel: "TestMode/Automatic/" ("Name Pattern") -> [_ _ w249 _ _]
          tunnel: T21 [{"Operation"=enum."Clear", "Color Box"=14013909}, {"Operation"=enum."Clear", "Color Box"=14013909}, {"Operation"=enum."Clear", "Color Box"=14013909}, {"Operation"=enum."Clear", "Color Box"=14013909}, {"Operation"=enum."Update", "Color Box"=14013909}, {"Operation"=enum."Update", "Color Box"=16777215}, {"Operation"=enum."Clear", "Color Box"=14013909}, {"Operation"=enum."Clear", "Color Box"=14013909}, {"Operation"=enum."Clear", "Color Box"=14013909}] -> [_ _ w242 _ w270]
          tunnel: w231 -> [_ _ w241 _ w269]
          tunnel: u32[] [15790320, 15790320, 15790320, 15790320, 16777215, 16777215, 15790320, 15790320, 15790320] -> [_ _ _ _ w275]
          tunnel: w229 -> [_ _ _ _ w263]
          tunnel: w226 -> [_ w236 _ _ _]
          frame "Custom", Default {
          }
          frame "Basic" {
            n110 = call <vilib>:"WPI_DashboardUpdateNames.vi"("Controls on Tab"=w236) -> ()  [unwired: 11 in]
          }
          frame "Test" {
            w248 = -2 ("Active Item:Row Number")
            n111 = Index Array(array=w242, index=w241) -> (element=w243:T24)
            n112 = Unbundle(w243) -> ("Operation"=w244:enum16{"Update", "Clear"}, "Color Box"=w245:u32)
            n113 = call <vilib>:"NT Read String.vi"("Name"="TestMode/TestName") -> ("String"=w239:string)  [unwired: 9 in, 1 out]
            n114 = call <vilib>:"NT Read and Format Entries as Tree.vi"("Operation"=w244, "Name Pattern"=w249, "Tree Refnum"=w250) -> ()  [unwired: 7 in, 2 out]
            n115 = case shown="\"\"" w239 {
              tunnel: "TestMode/TestProgress" ("Name") -> [w252 _]
              tunnel: "TestMode/TestProgressText" ("Name") -> [w251 _]
              frame Default {
                n116 = call <vilib>:"NT Read Number.vi"("Name"=w252) -> ("Numeric"=w253:dbl)  [unwired: 9 in, 1 out]
                n117 = call <vilib>:"NT Read String.vi"("Name"=w251) -> ("String"=w254:string)  [unwired: 9 in, 1 out]
                n118 = Bundle("Numeric"=w253, "String"=w254) -> (→"Progress":cluster{"Numeric":dbl, "String":string})  [unwired: 1 in]
              }
              frame "" {
                n119 = property on="Progress" class="Clust (strict)"("Visible"=FALSE) -> ()  [unwired: 2 in, 2 out]
                n120 = local write "Test Name"(u16 0) -> ()
              }
            }
            n121 = property on="Test Tree" class="Tree (strict)"("Active Item Row Number"=w248, "ActiveColNum"=w248, "CellBG"=w245, "Active Item Row Number"=-1 ("Active Item:Row Number"), "CellBG"=u32 5789784 ("Color Box")) -> ()  [unwired: 2 in, 2 out]
          }
          frame "Variables" {
            w260 = string[] ["CameraPublisher", "Usage", "DB"]  # Items to initially close
            n122 = First Call?() -> (First Call?: T/F=w261:bool)
            n123 = control-ref of="Tree"() -> (w262:refnum<vi>)
            n124 = Select(t=w260, s=w261, f=string[] []) -> (s? t:f=w258:string[])
            n125 = call <vilib>:"NT Read and Format Entries as Tree.vi"("Tags to  Close"=w258, "Tree Refnum"=w262) -> ()  [unwired: 8 in, 2 out]
          }
          frame "Commands" {
            w271 = u32 5789784 ("Color Box")
            w272 = T25 {"Row"=-1, "Column"=-2} ("Active Cell:Active Cell")
            w274 = T25 {"Row"=-2, "Column"=-2} ("Active Cell:Active Cell")
            n126 = Index Array(array=w275, index=w269) -> (element=w273:u32)
            n127 = Index Array(array=w270, index=w269) -> (element=w268:T24)
            n128 = Unbundle(w268) -> ("Operation"=w267:enum16{"Update", "Clear"})  [unwired: 1 out]
            n129 = local read "Command Selection"() -> (w266:i32)
            n130 = property on="Command Selection" class="MCListbox (strict)"("ActiveCell"=w274, "CellBG"=w273, "ActiveCell"=w272, "CellBG"=w271) -> ()  [unwired: 2 in, 2 out]
            n131 = call <vilib>:"WPI_DashboardUpdate RPC Info.vi"("Operation"=w267) -> ("update"=w265:bool, "commands"=w264:string[][])  [unwired: 9 in]
            n132 = property on="Command Selection" class="MCListbox (strict)"("ItemNames"=w264) -> ()  [unwired: 2 in, 2 out]
            n133 = property on="Command Params" class="Tbl (strict)"("Active Cell"=w274, "Cell BG Color"=w273, "Active Cell"=w272, "Cell BG Color"=w271) -> ()  [unwired: 2 in, 2 out]
            n134 = call <vilib>:"WPI_DashboardUpdate Command Params.vi"("Update"=w265, "NewVal"=w266, "Commands"=w264, "Param Tbl"=w263) -> ()  [unwired: 7 in, 1 out]
          }
        }
        n135 = call <vilib>:"Connextion Info.vi"() -> ("Connected"=→"NT Connection":bool)  [unwired: 10 in, 1 out]
      }
      event "Test Tree": Value Change {
        # "Show appropriate\ncontrols"
        n136 = event-data() -> ("CtlRef"=w280:refnum<vi>, "NewVal"=w278:string)  [unwired: 1 in]
        n137 = call <vilib>:"WPI_UtilitiesGetTreeIOName.vi"("NewVal"=w278, "TreeControl in"=w280) -> ("I/O Name"=w281:string)  [unwired: 9 in]
        n138 = case shown="\"Camera\"" w281 {
          selector: w281 -> [_ w288 _ w310 w319 _]
          tunnel: w278 -> [_ _ w307 w309 _ w326]
          tunnel: cluster{string[]}[] [{["640x480", "320x240", "160x120"]}, {["Auto", "Fixed indoor", "Fixed outdoor 1", "Fixed outdoor 2", "Fixed fluorescent 1", "Fixed fluorescent 2", "Hold current"]}, {["Auto", "Flicker-free 50 Hz", "Flicker-free 60 Hz", "Hold current"]}, {["None", "Prioritize frame rate", "Prioritize image quality"]}, {["Monochrome", "Color"]}] -> [_ _ _ _ _ w325]
          frame Default {
            w283 = FALSE ("Visible")
            w282 = FALSE ("Visible")
            n139 = property on="Motor" class="Clust (strict)"("Visible"=w282) -> ()  [unwired: 2 in, 2 out]
            n140 = property on="Test Ring" class="Ring (strict)"("Visible"=w282) -> ()  [unwired: 2 in, 2 out]
            n141 = property on="Rev/Fwd" class="Clust (strict)"("Visible"=w283) -> ()  [unwired: 2 in, 2 out]
            n142 = property on="On/Off" class="Bool (strict)"("Visible"=w283) -> ()  [unwired: 2 in, 2 out]
            n143 = property on="Test Slider" class="Slide (strict)"("Visible"=w283) -> ()  [unwired: 2 in, 2 out]
          }
          frame "Analog Out", "Motor", "PWM" {
            w289 = FALSE ("Visible")
            n144 = case shown="\"Analog Out\"" w288 {
              tunnel: [1.0 ("Value") -1.0 ("Value") 0.0 ("Value")] -> w287
              tunnel: [255.0 ("Value") 1.0 ("Value") 5.0 ("Value")] -> w286
              tunnel: [128.0 ("Value") 0.0 ("Value") 0.0 ("Value")] -> w285
              tunnel: [64.0 ("Value") 0.5 ("Value") 1.0 ("Value")] -> w284
              frame "PWM" {
              }
              frame "Motor", Default {
              }
              frame "Analog Out" {
              }
            }
            n145 = property on="Motor" class="Clust (strict)"("Visible"=TRUE) -> ()  [unwired: 2 in, 2 out]
            n146 = property on="Value" class="Slide (strict)"("Value"=w285, "Scale.Minimum"=w287, "Scale.Maximum"=w286, "Scale.Increment"=w284) -> ()  [unwired: 2 in, 2 out]
            n147 = property on="On/Off" class="Bool (strict)"("Visible"=w289) -> ()  [unwired: 2 in, 2 out]
            n148 = property on="Test Slider" class="Slide (strict)"("Visible"=w289) -> ()  [unwired: 2 in, 2 out]
            n149 = property on="Test Ring" class="Ring (strict)"("Visible"=w289) -> ()  [unwired: 2 in, 2 out]
            n150 = property on="Rev/Fwd" class="Clust (strict)"("Visible"=w289) -> ()  [unwired: 2 in, 2 out]
          }
          frame "Servo" {
            w305 = FALSE ("Visible")
            n151 = call <vilib>:"NT Read Number.vi"("Name"=w307) -> ("Numeric"=w306:dbl)  [unwired: 9 in, 1 out]
            n152 = property on="Test Slider" class="Slide (strict)"("Visible"=TRUE, "Scale.Maximum"=170.0 ("Scale.Range:Maximum")) -> ()  [unwired: 2 in, 2 out]
            n153 = local write "Test Slider"(w306) -> ()
            n154 = property on="Motor" class="Clust (strict)"("Visible"=w305) -> ()  [unwired: 2 in, 2 out]
            n155 = property on="Rev/Fwd" class="Clust (strict)"("Visible"=w305) -> ()  [unwired: 2 in, 2 out]
            n156 = property on="On/Off" class="Bool (strict)"("Visible"=w305) -> ()  [unwired: 2 in, 2 out]
            n157 = property on="Test Ring" class="Ring (strict)"("Visible"=w305) -> ()  [unwired: 2 in, 2 out]
          }
          frame "Relay", "Solenoid" {
            w308 = FALSE ("Visible")
            n158 = property on="Motor" class="Clust (strict)"("Visible"=w308) -> ()  [unwired: 2 in, 2 out]
            n159 = property on="Test Slider" class="Slide (strict)"("Visible"=w308) -> ()  [unwired: 2 in, 2 out]
            n160 = Search and Replace String(input string=w309, search string="/Value  **", replace string="/Direction") -> (result string=w315:string)  [unwired: 5 in, 3 out]
            n161 = property on="Test Ring" class="Ring (strict)"("Visible"=w308) -> ()  [unwired: 2 in, 2 out]
            n162 = call <vilib>:"NT Read String.vi"("Name"=w315) -> ("String"=w313:string)  [unwired: 9 in, 1 out]
            n163 = Equal?(x="Both directions", y=w313) -> (x = y?=w311:bool)
            n164 = Not(x=w311) -> (.not. x?=w312:bool)
            n165 = property on="Rev/Fwd" class="Clust (strict)"("Visible"=w311) -> ()  [unwired: 2 in, 2 out]
            n166 = property on="On/Off" class="Bool (strict)"("Visible"=w312, "Caption.Text"=w310) -> ()  [unwired: 2 in, 2 out]
          }
          frame "Compressor", "Digital Out" {
            w318 = FALSE ("Visible")
            # "Get direction and finish"
            n167 = property on="Motor" class="Clust (strict)"("Visible"=w318) -> ()  [unwired: 2 in, 2 out]
            n168 = property on="Test Slider" class="Slide (strict)"("Visible"=w318) -> ()  [unwired: 2 in, 2 out]
            n169 = property on="Test Ring" class="Ring (strict)"("Visible"=w318) -> ()  [unwired: 2 in, 2 out]
            n170 = property on="On/Off" class="Bool (strict)"("Visible"=TRUE, "Caption.Text"=w319) -> ()  [unwired: 2 in, 2 out]
            n171 = property on="Rev/Fwd" class="Clust (strict)"("Visible"=FALSE) -> ()  [unwired: 2 in, 2 out]
          }
          frame "Camera" {
            n172 = call <vilib>:"Get Last Path Segment.vi"("String in"=w326) -> ("String out"=w327:string)  [unwired: 10 in]
            n173 = property on="On/Off" class="Bool (strict)"("Visible"=FALSE) -> ()  [unwired: 2 in, 2 out]
            n174 = property on="Motor" class="Clust (strict)"("Visible"=FALSE) -> ()  [unwired: 2 in, 2 out]
            n175 = property on="Rev/Fwd" class="Clust (strict)"("Visible"=FALSE) -> ()  [unwired: 2 in, 2 out]
            n176 = case shown="\"White Balance  **\"" w327 {
              tunnel: w326 -> [w333 w342 w351 w360 w369 _ w375]
              tunnel: w325 -> [w331 w339 w348 w357 w366 _ _]
              frame "Size  **" {
                n177 = Index Array(array=w331) -> (element=w330:cluster{string[]})  [unwired: 1 in]
                n178 = call <vilib>:"NT Read String.vi"("Name"=w333) -> ("String"=w332:string)  [unwired: 9 in, 1 out]
                n179 = Unbundle(w330) -> (w328:string[])
                n180 = Match First String(2:w328, 3:w332) -> (0:w329:i32)  [unwired: 1 out]
                n181 = property on="Test Ring" class="Ring (strict)"("Value"=w329, "Strings []"=w328) -> ()  [unwired: 2 in, 2 out]
                n182 = property on="Test Ring" class="Ring (strict)"("Visible"=TRUE) -> ()  [unwired: 2 in, 2 out]
                n183 = property on="Test Slider" class="Slide (strict)"("Visible"=FALSE) -> ()  [unwired: 2 in, 2 out]
              }
              frame "White Balance  **" {
                n184 = Index Array(array=w339, index=1) -> (element=w340:cluster{string[]})
                n185 = call <vilib>:"NT Read String.vi"("Name"=w342) -> ("String"=w341:string)  [unwired: 9 in, 1 out]
                n186 = Unbundle(w340) -> (w337:string[])
                n187 = Match First String(2:w337, 3:w341) -> (0:w336:i32)  [unwired: 1 out]
                n188 = property on="Test Ring" class="Ring (strict)"("Value"=w336, "Strings []"=w337) -> ()  [unwired: 2 in, 2 out]
                n189 = property on="Test Ring" class="Ring (strict)"("Visible"=TRUE) -> ()  [unwired: 2 in, 2 out]
                n190 = property on="Test Slider" class="Slide (strict)"("Visible"=FALSE) -> ()  [unwired: 2 in, 2 out]
              }
              frame "Exposure  **" {
                n191 = Index Array(array=w348, index=2) -> (element=w349:cluster{string[]})
                n192 = call <vilib>:"NT Read String.vi"("Name"=w351) -> ("String"=w350:string)  [unwired: 9 in, 1 out]
                n193 = Unbundle(w349) -> (w345:string[])
                n194 = Match First String(2:w345, 3:w350) -> (0:w346:i32)  [unwired: 1 out]
                n195 = property on="Test Ring" class="Ring (strict)"("Value"=w346, "Strings []"=w345) -> ()  [unwired: 2 in, 2 out]
                n196 = property on="Test Ring" class="Ring (strict)"("Visible"=TRUE) -> ()  [unwired: 2 in, 2 out]
                n197 = property on="Test Slider" class="Slide (strict)"("Visible"=FALSE) -> ()  [unwired: 2 in, 2 out]
              }
              frame "Exposure Priority  **" {
                n198 = Index Array(array=w357, index=3) -> (element=w358:cluster{string[]})
                n199 = call <vilib>:"NT Read String.vi"("Name"=w360) -> ("String"=w359:string)  [unwired: 9 in, 1 out]
                n200 = Unbundle(w358) -> (w354:string[])
                n201 = Match First String(2:w354, 3:w359) -> (0:w355:i32)  [unwired: 1 out]
                n202 = property on="Test Ring" class="Ring (strict)"("Value"=w355, "Strings []"=w354) -> ()  [unwired: 2 in, 2 out]
                n203 = property on="Test Ring" class="Ring (strict)"("Visible"=TRUE) -> ()  [unwired: 2 in, 2 out]
                n204 = property on="Test Slider" class="Slide (strict)"("Visible"=FALSE) -> ()  [unwired: 2 in, 2 out]
              }
              frame "Color Enable  **" {
                n205 = Index Array(array=w366, index=4) -> (element=w367:cluster{string[]})
                n206 = call <vilib>:"NT Read String.vi"("Name"=w369) -> ("String"=w368:string)  [unwired: 9 in, 1 out]
                n207 = Unbundle(w367) -> (w363:string[])
                n208 = Match First String(2:w363, 3:w368) -> (0:w364:i32)  [unwired: 1 out]
                n209 = property on="Test Ring" class="Ring (strict)"("Value"=w364, "Strings []"=w363) -> ()  [unwired: 2 in, 2 out]
                n210 = property on="Test Ring" class="Ring (strict)"("Visible"=TRUE) -> ()  [unwired: 2 in, 2 out]
                n211 = property on="Test Slider" class="Slide (strict)"("Visible"=FALSE) -> ()  [unwired: 2 in, 2 out]
              }
              frame Default {
                n212 = property on="Test Ring" class="Ring (strict)"("Visible"=FALSE) -> ()  [unwired: 2 in, 2 out]
                n213 = property on="Test Slider" class="Slide (strict)"("Visible"=FALSE) -> ()  [unwired: 2 in, 2 out]
              }
              frame "Brightness  **", "Color Level  **", "Compression  **", "FPS  **", "Sharpness  **" {
                n214 = call <vilib>:"NT Read Number.vi"("Name"=w375) -> ("Numeric"=w374:dbl)  [unwired: 9 in, 1 out]
                n215 = local write "Test Slider"(w374) -> ()
                n216 = property on="Test Slider" class="Slide (strict)"("Visible"=TRUE, "Scale.Maximum"=100.0 ("Scale.Range:Maximum")) -> ()  [unwired: 2 in, 2 out]
                n217 = property on="Test Ring" class="Ring (strict)"("Visible"=FALSE) -> ()  [unwired: 2 in, 2 out]
              }
            }
          }
        }
        n218 = property on="Progress" class="Clust (strict)"("Visible"=FALSE) -> ()  [unwired: 2 in, 2 out]
      }
      event "Test Name": Mouse Enter {
        # "Populate the ring with the list of tests"
        n219 = event-data() -> ()  [unwired: 1 in, 1 out]
        n220 = call <vilib>:"NT Read String Array.vi"("Name"="TestMode/TestList") -> ("String Array"=w383:string[])  [unwired: 9 in, 1 out]
        n221 = Build Array (concatenate)("Select the test to run...", w383) -> (w382:string[])
        n222 = property on="Test Name" class="Ring (strict)"("Strings []"=w382) -> ()  [unwired: 2 in, 2 out]
      }
      event "Test Name": Value Change {
        w385 = FALSE ("Visible")
        # "Tell the robot the test name to run"
        n223 = event-data() -> ("NewVal"=w389:u16)  [unwired: 1 in]
        n224 = property on="Test Name" class="Ring (strict)"() -> ("Strings []"=w390:string[])  [unwired: 2 in, 2 out]
        n225 = local write "Progress"(T6 {"Test Progress"=0, "Test Progress Text"=""} ("Progress")) -> ()
        n226 = Index Array(array=w390, index=w389) -> (element=w388:string)
        n227 = call <vilib>:"NT Write String.vi"("String"=w388, "Name"="TestMode/TestName") -> ()  [unwired: 9 in, 1 out]
        n228 = property on="Progress" class="Clust (strict)"("Visible"=TRUE) -> ()  [unwired: 2 in, 2 out]
        n229 = property on="Motor" class="Clust (strict)"("Visible"=w385) -> ()  [unwired: 2 in, 2 out]
        n230 = property on="Test Slider" class="Slide (strict)"("Visible"=w385) -> ()  [unwired: 2 in, 2 out]
        n231 = property on="On/Off" class="Bool (strict)"("Visible"=w385) -> ()  [unwired: 2 in, 2 out]
        n232 = property on="Rev/Fwd" class="Clust (strict)"("Visible"=w385) -> ()  [unwired: 2 in, 2 out]
        n233 = property on="Test Ring" class="Ring (strict)"("Visible"=w385) -> ()  [unwired: 2 in, 2 out]
      }
      event "Select Auto": Mouse Enter {
        # "Populate the combo box with the list of autonomous options"
        n234 = event-data() -> ()  [unwired: 1 in, 1 out]
        n235 = call <vilib>:"NT Read String Array.vi"("Name"="Auto List") -> ("String Array"=w392:string[])  [unwired: 9 in, 1 out]
        n236 = property on="Select Auto" class="CmbBox"("Strings[]"=w392) -> ()  [unwired: 2 in, 2 out]
      }
      event "Select Auto": Value Change {
        # "User modified the Auto Selection. Write to NT variable so robot knows."
        n237 = event-data() -> ("NewVal"=w395:string)  [unwired: 1 in]
        n238 = call <vilib>:"NT Write String.vi"("String"=w395, "Name"="Auto Selector") -> ()  [unwired: 9 in, 1 out]
      }
      event "Command Selection": Value Change {
        # "Get the params and show in table"
        n239 = event-data() -> ("NewVal"=w401:i32)  [unwired: 1 in]
        n240 = property on="Command Selection" class="MCListbox (strict)"() -> ("ItemNames"=w399:string[][])  [unwired: 2 in, 2 out]
        n241 = call <vilib>:"WPI_DashboardUpdate Command Params.vi"("NewVal"=w401, "Commands"=w399, "Param Tbl"=w400) -> ()  [unwired: 8 in, 1 out]
      }
      event "Execute Command": Value Change {
        # "Started one, Unique ID holds\nresponse"
        n242 = event-data() -> ()  [unwired: 1 in, 1 out]
        n243 = property on="Command Selection" class="MCListbox (strict)"() -> ("ItemNames"=w412:string[][])  [unwired: 2 in, 2 out]
        n244 = Index Array(array=w412, index (row)="Command Selection", index (col)=0) -> (element=w410:string)
        n245 = call <vilib>:"Invoke Commands.vi"("Command Params"="Command Params", "Function Name"=w410) -> ("Params"=w406:u8, "Started"=w405:bool)  [unwired: 7 in, 1 out]
        n246 = Array Subset(array="Command Params", length (row)=w406) -> (w407:string[][])  [unwired: 3 in]
        n247 = Select(t="Executing" ("Cmd Status"), s=w405, f="" ("Cmd Status")) -> (s? t:f=→"Cmd Status":string)
      }
      event "Command Selection": Double Click {
        n248 = event-data() -> ("Row"=w420:i32)  [unwired: 1 in]
        n249 = property on="Command Selection" class="MCListbox (strict)"() -> ("ItemNames"=w423:string[][])  [unwired: 2 in, 2 out]
        n250 = local read "Command Params"() -> (w419:string[][])
        n251 = Index Array(array=w423, index (row)=w420, index (col)=0) -> (element=w421:string)
        n252 = call <vilib>:"Invoke Commands.vi"("Command Params"=w419, "Function Name"=w421) -> ("Params"=w418:u8, "Started"=w413:bool)  [unwired: 7 in, 1 out]
        n253 = Array Subset(array=w419, length (row)=w418) -> (w417:string[][])  [unwired: 3 in]
        n254 = Select(t="Executing" ("Cmd Status"), s=w413, f="" ("Cmd Status")) -> (s? t:f=w414:string)
        n255 = local write "Cmd Status"(w414) -> ()
      }
      event "CheckList": Double Click {
        # "Shift clears all"
        # "Update symbols on the listbox"
        n256 = event-data() -> ("PlatMods.Shift"=w425:bool, "Row"=w427:i32)  [unwired: 1 in]
        n257 = case shown="True" w425 {
          tunnel: w427 -> [w431 _]
          tunnel: 1 -> [w430 _]
          frame False {
            n258 = property on="CheckList" class="LstBox (strict)"() -> ("Item Symbols"=w429:i32[])  [unwired: 2 in, 2 out]
            n259 = Replace Array Subset(array=w429, new element=w430, index=w431) -> (w428:i32[])
            n260 = property on="CheckList" class="LstBox (strict)"("Item Symbols"=w428) -> ()  [unwired: 2 in, 2 out]
          }
          frame True {
            w432 = 0 ("Top Row")
            n261 = property on="CheckList" class="LstBox (strict)"() -> ("Number of Rows"=w434:u32)  [unwired: 2 in, 2 out]
            n262 = Initialize Array(0, w434) -> (w433:i32[])
            n263 = property on="CheckList" class="LstBox (strict)"("Top Row"=w432, "Value"=w432, "Item Symbols"=w433) -> ()  [unwired: 2 in, 2 out]
          }
        }
      }
      event "CheckList": Key Down {
        # "Update symbols on the listbox\nLeft and right keys check and uncheck"
        n264 = event-data() -> ("VKey"=w438:T22)  [unwired: 1 in]
        n265 = case shown="\"Left\", \"Right\"" w438 {
          selector: w438 -> [w443 _]
          tunnel: eventvkey."Left" ("VKey") -> [w441 _]
          frame "Left", "Right" {
            n266 = Equal?(x=w441, y=w443) -> (x = y?=w442:bool)
            n267 = Select(t=0, s=w442, f=1) -> (s? t:f=w444:i32)
            n268 = property on="CheckList" class="LstBox (strict)"() -> ("Item Symbols"=w447:i32[])  [unwired: 2 in, 2 out]
            n269 = Replace Array Subset(array=w447, new element=w444, index="CheckList") -> (w446:i32[])
            n270 = property on="CheckList" class="LstBox (strict)"("Item Symbols"=w446) -> ()  [unwired: 2 in, 2 out]
          }
          frame Default {
          }
        }
      }
      event "Motor.Enable": Value Change {
        # "When the test mode otor enable helper is set, update that\ntree row item's value"
        n271 = event-data() -> ("NewVal"=w453:bool)  [unwired: 1 in]
        n272 = Unbundle("Motor") -> ("Value"=w452:dbl)  [unwired: 1 out]
        n273 = Select(t=w452, s=w453, f=0.0) -> (s? t:f=w450:dbl)
        n274 = call <vilib>:"NT Write Number.vi"("Numeric"=w450, "Name"=w449) -> ()  [unwired: 9 in, 1 out]
      }
      event "Test Slider": Value Change {
        # "When the test mode slider helper is set, update that\ntree row item's value"
        n275 = event-data() -> ("NewVal"=w456:dbl)  [unwired: 1 in]
        n276 = call <vilib>:"NT Write Number.vi"("Numeric"=w456, "Name"=w457) -> ()  [unwired: 9 in, 1 out]
      }
      event "On/Off": Value Change {
        # "When the test mode on/off helper value is set, update that\ntree row item's value"
        n277 = event-data() -> ("NewVal"=w461:bool)  [unwired: 1 in]
        n278 = Boolean To (0,1)(Boolean=w461) -> (0, 1=w460:i16)
        n279 = call <vilib>:"NT Write Number.vi"("Numeric"=w460, "Name"=w459) -> ()  [unwired: 9 in, 1 out]
      }
      event "Rev/Fwd": Value Change {
        # "When the test mode helper value for relays is set, update that\ntree row item's value"
        n280 = event-data() -> ("NewVal.Forward"=w469:bool, "NewVal.Reverse"=w468:bool)  [unwired: 1 in]
        n281 = Boolean To (0,1)(Boolean=w469) -> (0, 1=w465:i16)
        n282 = Boolean To (0,1)(Boolean=w468) -> (0, 1=w467:i16)
        n283 = Negate(x=w467) -> (-x=w466:i16)
        n284 = Add(x=w465, y=w466) -> (x+y=w464:i16)
        n285 = call <vilib>:"NT Write Number.vi"("Numeric"=w464, "Name"=w463) -> ()  [unwired: 9 in, 1 out]
      }
      event "Test Ring": Value Change {
        # "When a test mode helper value is selected from the ring,\nset the tree item's variable to the string value"
        n286 = event-data() -> ("NewVal"=w473:u16)  [unwired: 1 in]
        n287 = property on="Test Ring" class="Ring (strict)"() -> ("Strings []"=w474:string[])  [unwired: 2 in, 2 out]
        n288 = Index Array(array=w474, index=w473) -> (element=w472:string)
        n289 = call <vilib>:"NT Write String.vi"("String"=w472, "Name"=w471) -> ()  [unwired: 9 in, 1 out]
      }
      event "Rec Mode": Value Change {
        # "Update globals for recording mode and path to read log from.\nClear when logging and let NetworkTables set path for vision to\nuse."
        n290 = event-data() -> ("NewVal"=w485:enum32{"Stop", "Record", "Playback"})  [unwired: 1 in]
        n291 = global write "WPI_DashboardLogging Global.vi" "Logging Filename"(path "") -> ()
        n292 = global write "WPI_DashboardLogging Global.vi" "Recording"(w485) -> ()
        n293 = case shown="\"Playback\"" w485 {
          tunnel: w484 -> [_ w487 w496]
          tunnel: [_ _ w495] -> w482
          tunnel: [_ _ w494] -> _
          tunnel: w480 -> [_ _ w492]
          tunnel: cluster{i32, i32} {-250, 170} -> [_ _ w491]
          tunnel: [_ _ T23 {"Image Size"=TRUE, "Image Type"=TRUE, "Pixel Value"=TRUE, "ROI Information"=TRUE, "Zoom Factor"=FALSE} ("Image Information Shown:All Elements")] -> w475
          tunnel: [_ _ TRUE ("Zoom Factor")] -> w476
          tunnel: w478 -> [_ _ w488]
          frame Default {
          }
          frame "Stop", "Record" {
            # "Place Window too"
            n294 = invoke class="VI" method="FP.Close"(reference=w487) -> (reference out=w486:refnum<vi>)  [unwired: 2 in, 2 out]
            n295 = invoke class="VI" method="Abort VI"(reference=w486) -> ()  [unwired: 2 in, 3 out]
          }
          frame "Playback" {
            n296 = call "Open Playback Panel.vi"("Offset"=w491, "DB VI Ref"=w492, "Playback in"=w496) -> ("Playback out"=w493:refnum<vi>)  [unwired: 8 in]
            n297 = register-events(w493, w488) -> (reference out=w495:refnum<event-registration>, error out=w494:errorcluster)  [unwired: 2 in]
          }
        }
        n298 = property on="Camera Image Right" class="ImageControl"("Image Information Shown"=w475, "Image Information Visible"=w476) -> ()  [unwired: 2 in, 2 out]
        n299 = property on="Camera Image" class="ImageControl"("Image Information Shown"=w475, "Image Information Visible"=w476) -> ()  [unwired: 2 in, 2 out]
        n300 = call <vilib>:"WPI_DashboardNT Log FieldName Cache.vi"("Operation"=enum16{"Lookup/Add", "Index", "Clear"}."Clear") -> ()  [unwired: 8 in, 3 out]
      }
      event Panel Close {
        w498 = enum32{"Stop", "Record", "Playback"}."Stop" ("Rec Mode")
        # "Playback window has been closed, abort"
        n301 = event-data() -> ()  [unwired: 1 in, 4 out]
        n302 = local write "Rec Mode"(w498) -> ()
        n303 = global write "WPI_DashboardLogging Global.vi" "Recording"(w498) -> ()
      }
      event Panel Close {
        # "Abort playback window and ourself"
        n304 = event-data() -> ()  [unwired: 1 in, 4 out]
        n305 = invoke class="VI" method="FP.Close"(reference=w502) -> (reference out=w501:refnum<vi>)  [unwired: 2 in, 2 out]
        n306 = invoke class="VI" method="Abort VI"(reference=w501) -> (error out=w500:errorcluster)  [unwired: 2 in, 2 out]
        n307 = invoke class="VI" method="Abort VI"(error in=w500) -> ()  [unwired: 2 in, 3 out]
      }
      event User Event {
        n308 = event-data() -> ("IDs"=w509:cluster{"RPC field ID":u16, "Unique ID":u16}, "String"=w508:string)  [unwired: 1 in]
        n309 = Bundle("IDs"=w509, "String"=w508) -> (w507:T9)  [unwired: 1 in]
        n310 = call <vilib>:"Retrieve RPC Response.vi"("RPC Response"=w507) -> ("Output"=w505:string[][])  [unwired: 10 in]
        n311 = Build Array (concatenate)(w503, w505) -> (w504:string[][])
        n312 = local write "Command Params"(w504) -> ()
        n313 = local write "Cmd Status"("" ("Cmd Status")) -> ()
      }
      event "Tree": Double Click {
        n314 = event-data() -> ("PlatMods"=w515:T26, "Tag"=w512:string)  [unwired: 1 in]
        n315 = Unbundle(w515) -> ("Shift"=w514:bool)  [unwired: 4 out]
        n316 = String Subset(string=w512, length (rest)=1 ("length (rest)")) -> (substring=w511:string)  [unwired: 1 in]
        n317 = Not(x=w514) -> (.not. x?=w513:bool)
        n318 = case shown="\"/\"" w511 {
          tunnel: w512 -> [_ w518]
          tunnel: w513 -> [_ w517]
          frame Default {
          }
          frame "/" {
            n319 = call <vilib>:"NT Update Persistence.vi"("Persistence"=w517, "Name"=w518) -> ()  [unwired: 9 in, 1 out]
          }
        }
      }
    }
  }
  n320 = while {
    tunnel: w90 -> [w520]
    i -> [w523]
    stop <- FALSE stop-if-true
    n321 = Wait (ms)(milliseconds to wait=u32 100) -> ()  [unwired: 1 out]
    n322 = case shown="\"Playback\"" "Rec Mode" {
      tunnel: w523 -> [_ _ w538]
      tunnel: [u32 2829099 ("Base Color") u32 11141120 ("Target Color") w527] -> w519
      frame "Stop", Default {
        # "Reset the color, extra updates don't cost much"
      }
      frame "Record" {
      }
      frame "Playback" {
        # "Playback"
        n323 = Quotient & Remainder(x=w538, y=u32 50 ("milliseconds to wait")) -> (x-y*floor(x/y)=w534:u32)  [unwired: 1 out]
        n324 = Divide(x=w534, y=u32 50 ("milliseconds to wait")) -> (x/y=w531:dbl)
        n325 = Multiply(x=6.283185307179586, y=w531) -> (x*y=w536:dbl)
        n326 = Sine(x=w536) -> (sin(x)=w535:dbl)
        n327 = Absolute Value(x=w535) -> (abs(x)=w528:dbl)
        n328 = call "Interpolate RGB Color.vi"("Proportion"=w528, "Target Color"=u32 30976, "Base Color"=u32 2829099) -> ("Result Color"=w527:u32)  [unwired: 8 in]
      }
    }
    n329 = property class="Pane"(reference=w520, "PaneColor"=w519) -> ()  [unwired: 1 in, 2 out]
  }
  n330 = local write "Dashboard Tab"(T2."Drive" ("Dashboard Tab")) -> ()
  n331 = property on="On/Off" class="Bool (strict)"("Visible"=w61) -> ()  [unwired: 2 in, 2 out]
  n332 = property on="Motor" class="Clust (strict)"("Visible"=w61) -> ()  [unwired: 2 in, 2 out]
  n333 = property on="Progress" class="Clust (strict)"("Visible"=w61) -> ()  [unwired: 2 in, 2 out]
  n334 = property on="Test Ring" class="Ring (strict)"("Visible"=w61) -> ()  [unwired: 2 in, 2 out]
  n335 = property on="Rev/Fwd" class="Clust (strict)"("Visible"=w61) -> ()  [unwired: 2 in, 2 out]
  n336 = while {
    tunnel: u16 1741 ("timeout ms (25000)") -> [w540]
    stop <- FALSE stop-if-true
    n337 = TCP Create Listener(10:w540) -> (0:w539:errorcluster, 3:w541:refnum<k5>)  [unwired: 4 in, 1 out]
    n338 = case shown="No Error" w539 {
      selector: w539 -> [w543 _]
      tunnel: w541 -> [w544 _]
      frame No Error {
        n339 = while {
          tunnel: w544 -> [w547]
          tunnel: w543 -> [w546]
          stop <- FALSE stop-if-true
          n340 = TCP Wait On Listener(8:w546, 11:w547) -> (0:w548:errorcluster, 4:w549:refnum<k5>)  [unwired: 2 in, 3 out]
          n341 = local write "TCP"(w549) -> ()
          n342 = case shown="No Error" w548 {
            frame No Error {
            }
            frame Error {
              n343 = Wait (ms)(milliseconds to wait=u32 1000) -> ()  [unwired: 1 out]
            }
          }
        }
      }
      frame Error {
        n344 = Wait (ms)(milliseconds to wait=u32 1000) -> ()  [unwired: 1 out]
      }
    }
  }
  n345 = local write "Command Selection"(u16 0 ("milliseconds to wait")) -> ()
  n346 = local write "Command Params"(string[][] [] ("Command Params")) -> ()
  n347 = global write "WPI_DashboardLogging Global.vi" "Recording"(w84) -> ()
  n348 = local write "Rec Mode"(w84) -> ()
  n349 = call <vilib>:"NT Write String.vi"("String"="Select Auto", "Name"="Auto Selector") -> ()  [unwired: 9 in, 1 out]
  n350 = property on="Calibrate?" class="Bool (strict)"("BoolText.FontBold"=TRUE ("Boolean Text.Font:Bold"), "BoolText.TextColor"=u32 16711680, "BoolText.FontSize"=u32 32 ("Boolean Text.Font:Size"), "Label.FontBold"=TRUE ("Boolean Text.Font:Bold"), "Label.TextColor"=u32 16773632, "Label.FontSize"=u32 24 ("Boolean Text.Font:Size")) -> ()  [unwired: 2 in, 2 out]
  n351 = property on="PickUp/DropOff" class="Str"("Text.FontBold"=TRUE ("Text.Font:Bold"), "Label.Visible"=TRUE, "Text.FontSize"=u32 64 ("Text.Font:Size")) -> ()  [unwired: 2 in, 2 out]
  n352 = property on="ElevBasePos" class="Str"("Text.FontBold"=TRUE ("Text.Font:Bold"), "Label.Visible"=TRUE, "Text.FontSize"=u32 64 ("Text.Font:Size")) -> ()  [unwired: 2 in, 2 out]
  n353 = property on="SwerveMode" class="Str"("Text.FontBold"=TRUE ("Text.Font:Bold"), "Label.Visible"=TRUE, "Text.FontSize"=u32 64 ("Text.Font:Size")) -> ()  [unwired: 2 in, 2 out]
  n354 = property on="Robot Front" class="Bool (strict)"("BoolText.FontBold"=TRUE ("Boolean Text.Font:Bold"), "BoolText.TextColor"=u32 6618880, "BoolText.FontSize"=u32 32 ("Boolean Text.Font:Size"), "Label.FontBold"=TRUE ("Boolean Text.Font:Bold"), "Label.TextColor"=u32 3381759, "Label.FontSize"=u32 24 ("Boolean Text.Font:Size")) -> ()  [unwired: 2 in, 2 out]
  n355 = property on="Hatch Position" class="Bool (strict)"("BoolText.FontBold"=TRUE ("Boolean Text.Font:Bold"), "BoolText.FontSize"=u32 24 ("Boolean Text.Font:Size"), "Label.FontBold"=TRUE ("Boolean Text.Font:Bold"), "Label.FontSize"=u32 24 ("Boolean Text.Font:Size")) -> ()  [unwired: 2 in, 2 out]
